vi "x502_recv_out_cycle.vi"() -> ()   [LabVIEW 2010]
uses:
  <vilib>/Waveform/DWDTOps.llb/DWDT Binary U32 to Digital.vi
panel:
  in  "Частота сигнала (Гц)":dbl=50.0 min=1.0 max=500000.0
  in  "Смещение сигнала":dbl min=-5.0 max=5.0 format="%.2f"
  in  "Амплитуда сигнала":dbl=5.0 min=0.0 max=5.0 format="%.2f"
  in  "Подключение по IP":bool
  in  "IP Addr":string="192.168.0.1"
  out "MCU ver":string
  in  "START":bool
  in  "Список устройств USB/PCIe":u16(ring)
  out "Mixed Signal Graph":T1(graph)
  in  "Логические каналы":T2(array[cluster])=[{"PhyCh"=1, "Avg"=1, "Mode"=1, "Range"=0}, {"PhyCh"=2, "Avg"=1, "Mode"=1, "Range"=0}, {"PhyCh"=3, "Avg"=1, "Mode"=1, "Range"=0}] {"Range" items=["10 В", "5 В", "2 В", "1 В", "0.5 В", "0.2 В"]; "Mode" items=["С общей землей", "Дифференциальный", "Измерение нуля"]; "Avg" max=255 step=1; "PhyCh" min=1 max=32 step=1}
  in  "Отображать за время":dbl=250.0 min=10.0 step=1.0
  in  "stop":bool
  out "Установленная частота синхронного ввода DIN":dbl=2.0 min=2.0 max=2000000.0 format="%#_8f"
  in  "Частота синхронного ввода DIN":dbl=20000.0 min=1.0 max=2000000.0 format="%#_8f"
  out "FPGA Ver":string
  in  "Количество каналов":u32=3 min=1 max=3
  out "Установленная частота на канал":dbl=2.0 min=2.0 max=2000000.0 format="%#_8f"
  out "Установленная частота сбора":dbl=2.0 min=2.0 max=2000000.0 format="%#_8f"
  in  "Частота сбора на канал":dbl=2000000.0 min=2.0 max=2000000.0 format="%#_8f"
  in  "Частота сбора (Гц)":dbl=2000000.0 min=2.0 max=2000000.0 format="%#_8f"
  out "PldaVer":u8
  out "Serial":string
  out "Name":string
  # "Информация о плате"
  # "Настройки модуля"
  # "Устанавливаемое"
  # "Установленное"
  # "Вывод на ЦАП"
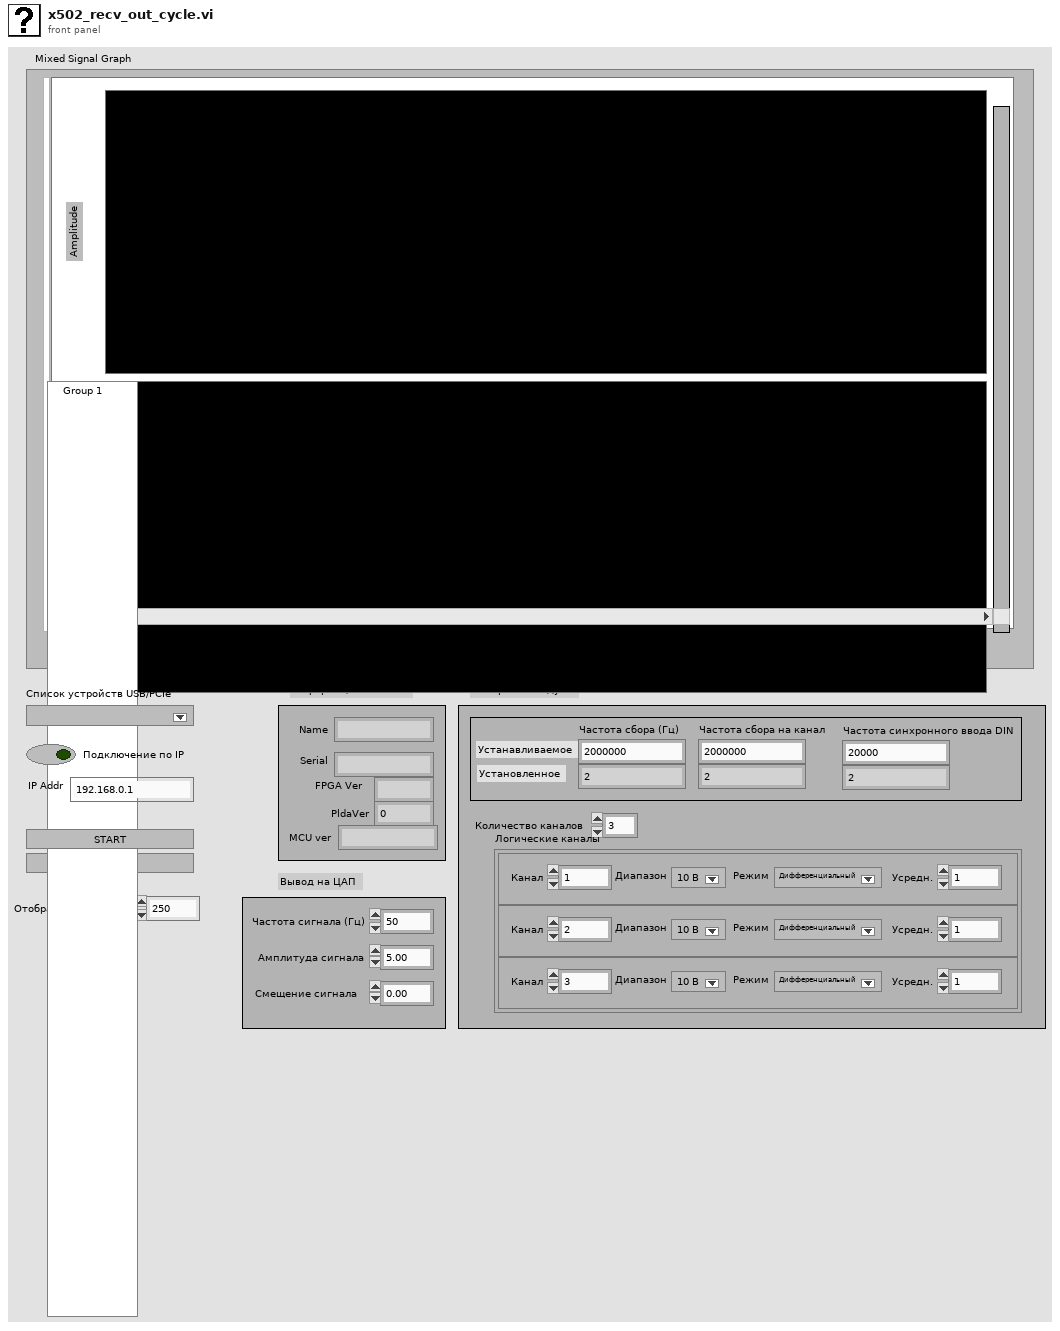
[diagram p1: front panel]
types:
  T1 = cluster{"Dynamic Data Type":dynamicdata, "digital waveform":digitalwaveform}
  T2 = cluster{"PhyCh":u32, "Avg":u32, "Mode":u32, "Range":u32}[]
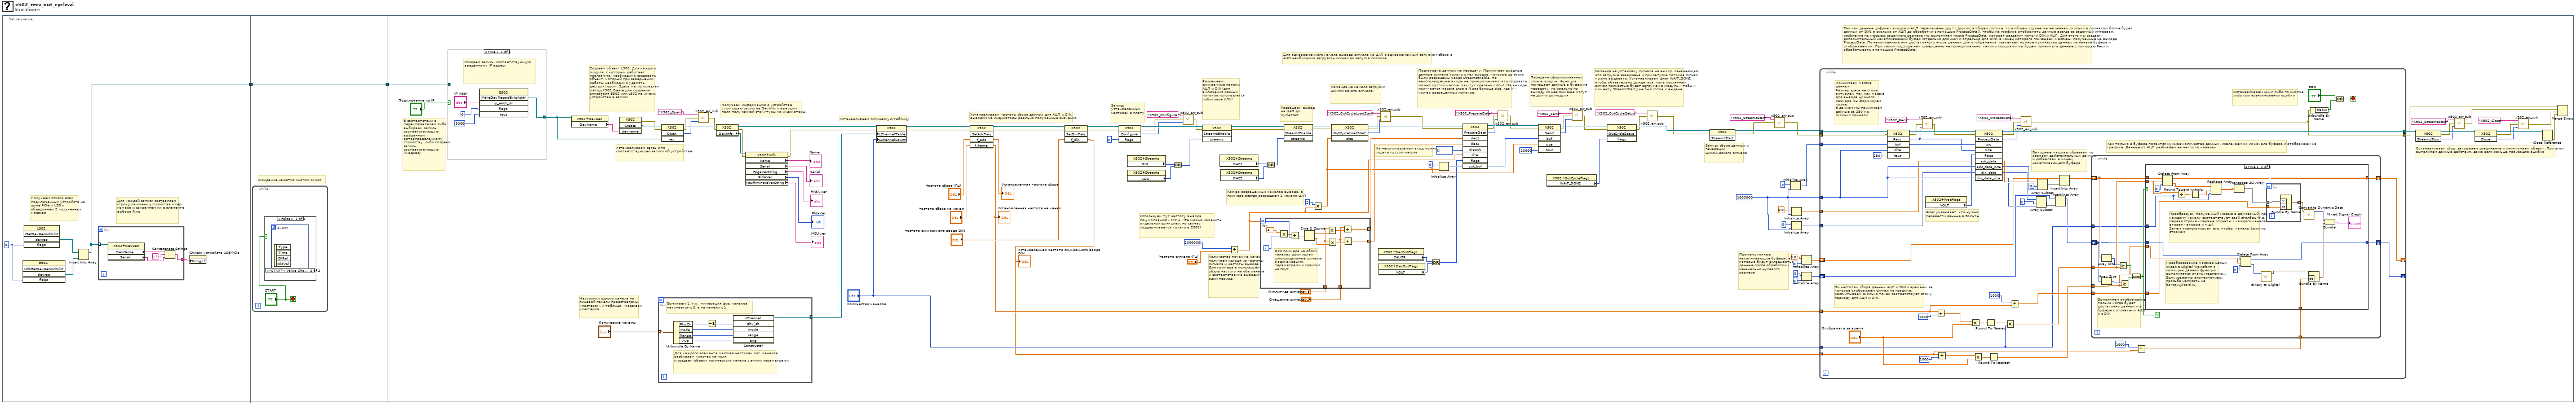
[diagram p0: block diagram]
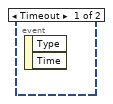
[diagram p2: hidden frame]
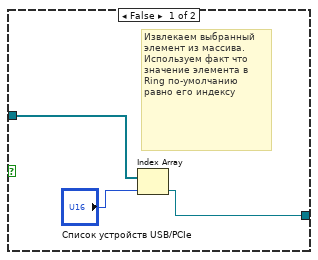
[diagram p5: hidden frame]
diagram:
  n1 = flat-sequence {
    tunnel: [w3] -> w1
    tunnel: [w13] -> w2
    tunnel: w1 -> [w13]
    tunnel: w2 -> [w94]
    frame #0 {
      w5 = 0
      # "Для каждой записи составляем строку из имени устройства и сер. номера и сохраняем их в элементе выбора Ring"
      # "Получаем списко всех подключенных устройств на шине PCIe и USB и объединяем 2 полученных массива"
      n2 = invoke class="E502" method="UsbGetDevRecordsList"("flags"=w5) -> ("devrec"=w6:refnum<k24>[])  [unwired: 4 in, 4 out]
      n3 = invoke class="L502" method="GetDevRecordsList"("flags"=w5) -> ("devrec"=w7:refnum<k24>[])  [unwired: 4 in, 4 out]
      n4 = Insert Into Array(array=w7, new element=w6) -> (w3:refnum<k24>[])  [unwired: 1 in]
      n5 = for {
        tunnel: [w9] -> w4 mode=indexing
        tunnel: w3 -> [w8] mode=indexing
        n6 = property class="X502+DevRec"(reference=w8) -> ("DevName"=w12:string, "Serial"=w10:string)  [unwired: 1 in, 2 out]
        n7 = Concatenate Strings(w12, ", ", w10) -> (w9:string)
      }
      n8 = property on="Список устройств USB/PCIe" class="Ring (strict)"("Strings []"=w4) -> ()  [unwired: 2 in, 2 out]
    }
    frame #1 {
      # "Ожидание нажатия кнопки START"
      n9 = while {
        stop <- "START" stop-if-true
        n10 = case shown="False" "START" {
          frame False {
            n11 = event shown="[1] \"START\": Value Change" {
              selector: _ -> [_ _]
              dyn-events: _ -> [_ _]
              timeout: _ -> [_ _]
              event Timeout {
                n12 = event-data() -> ()  [unwired: 1 in, 2 out]
              }
              event "START": Value Change {
                n13 = event-data() -> ()  [unwired: 1 in, 4 out]
              }
            }
          }
          frame True {
          }
        }
      }
    }
    frame #2 {
      w86 = u32 1000000 ("element")
      # "Останавливаем сбор, закрываем соединение и уничтожаем объект. При этом выполняем данные действия, даже если раньше произошла ошибка"
      # "Команда на установку сигнала на выход, означающая, что загрузка завершена и при запуске потоков сигнал можно выдавать. Устанавливаем флаг WAIT_DONE, чтобы обязательно дождаться, пока посланный сигнал полностью будет загружен в модуль, чтобы к моменту StreamsStart уже был готов к выдаче"
      # "Передача сформированных слов в модуль. Функция помещает данные в буфер на передачу, но раельно по выходу из нее они еще могут не дойти до модуля"
      # "Подготовка данных на передачу. Принимает входные данные сигнала только с тех входов, которые до этого были разрешены через StreamsEnable. На неиспользуемые входы не принципиально, что подовать, можно пустой массив, как тут сделано с dout. На выходе получается массив слов в N раз больше size, где N - кол-во разрешенных потоков."
      # "Команда на начало загрузки циклического сигнала."
      # "Для одновременного начала вывода сигнала на ЦАП с одновременным запуском сбора с АЦП необходимо загрузить сигнал до запуска потоков."
      # "На неиспользуемый вход можно подать пустой массив"
      # "Кол-во разрешенных каналов вывода. В примере всегда разрешаем 2 канала ЦАП"
      # "Количество точек на канал получаем исходя из частоты сигнала и частоты вывода. Для примера в используем обзую частоту на оба канала и соответственно выводим один период"
      # "Используем тут частоту вывода по-умолчанию - 1МГц . (Ее можно изменить отдельной функцией, но сейчас поддерживается только в E502)"
      # "Разрешаем вывод на ЦАП до CycleStart"
      # "Так как данные цифроых входов и АЦП перемешены друг с другом в общем потоке, то в общем случае мы не значем сколько в принятом блоке будет данных от DIN, а сколько от АЦП до обработки с помощью ProcessData(). Чтобы на графике отображать данные всегда за заданный интервал, разбиение на массивы заданного размера мы выполняем после ProcessData, которая разделит потоки DIN и АЦП. Для этого мы создаем дополнительный накапливающий буфер (отдельно для АЦП и отдельно для DIN), в конец которого помещаем массивы, полученные на выходе ProcessData. По накоплению в них достаточного числа данных для отображения  извлекаем нужное количество данных из начала буфера и отображаем их. При таком подходе нам совершенно не принципиально, какими порциями мы будем принимать данные с помощью Recv и обрабатывать с помощью ProcessData."
      # "Промежуточные накапливающие буферы, в которые будут складываться данные после обработки - изначально нулевого размера"
      # "Запуск сбора данных и генерации циклического сигнала"
      # "Разрешаем синхронные потоки АЦП и DIN (для включения разных потоков используется побитовое ИЛИ)"
      # "В соответствии с переключателем либо выбираем запись, соответствующую выбранном автоопределенному стройству, либо создаем запись, соответствующую IP-адресу"
      # "Запись установленных настроек в плату"
      # "Устанавливаем частоты сбора данных для АЦП и DIN,\nвыводим на индикаторы реально полученные значения"
      # "Устанавливаем логическую таблицу"
      # "Настройки одного канала на лицевой панели представлены кластером. А таблица - массивом кластеров."
      # "Создаем объект L502. Для каждого модуля, с которым работает программа, необходимо создавать объект, который при завершении работы необходимо удалять деструктором. Здесь мы используем метод X502.Create для создания описателя E502 или L502 по имени устройства в записи"
      # "Получаем информацию о устройстве \nс помощью свойства DevInfo и выводим\nполя полученной стркутуры на индикаторы"
      # "Устанавливаем связь с по соответствующей записи об устройстве"
      n14 = case shown="True" "Подключение по IP" {
        tunnel: w94 -> [w242 _]
        tunnel: [w240 w243] -> w93
        frame False {
          # "Извлекаем выбранный элемент из массива. Используем факт что значение элемента в Ring по-умолчанию равно его индексу"
          n15 = Index Array(array=w242, index="Список устройств USB/PCIe") -> (element=w240:refnum<k24>)
        }
        frame True {
          # "Создаем запись, соответствующую введенному IP адресу"
          n16 = invoke class="E502" method="MakeDevRecordByIpAddr"("ip_addr_str"="IP Addr", "flags"=0, "tout"=5000) -> ("MakeDevRecordByIpAddr"=w243:refnum<k24>)  [unwired: 3 in, 5 out]
        }
      }
      n17 = property class="X502+DevRec"(reference=w93) -> ("DevName"=w114:string)  [unwired: 1 in, 2 out]
      n18 = invoke class="X502" method="Create"("devname"=w114) -> (error out=w113:errorcluster, "Create"=w115:refnum<k24>)  [unwired: 3 in, 2 out]
      n19 = for {
        tunnel: "Логические каналы" -> [w253] mode=indexing
        tunnel: [w247] -> w131 mode=indexing
        # "Вычитаем 1, т.к.  нумерация физ. каналов начинается с 0, а на панели с 1"
        # "Для каждого элемента массива настроек лог. каналов разбиваем кластер на поля\nи создаем объект логического канала с этими параметрами"
        n20 = Unbundle By Name(w253) -> ("PhyCh"=w252:u32, "Mode"=w250:u32, "Range"=w249:u32, "Avg"=w248:u32)
        n21 = Decrement(x=w252) -> (x-1=w251:u32)
        n22 = constructor class="X502+LChannel"("phy_ch"=w251, "mode"=w250, "range"=w249, "avg"=w248) -> (reference out=w247:refnum<k24>)  [unwired: 3 in, 6 out]
      }
      n23 = invoke class="X502" method="Open"(reference=w115, error in=w113, "rec"=w93) -> (reference out=w116:refnum<k24>, error out=w111:errorcluster, "Open"=w112:i32)  [unwired: 1 in, 1 out]
      n24 = call "x502_err_sub.vi"("Error code"=w112, "error in (no error)"=w111, "Error descr"="X502_Open ") -> ("error out"=w109:errorcluster)
      n25 = property class="X502"(reference=w116, error in=w109) -> (reference out=w117:refnum<k24>, error out=w107:errorcluster, "DevInfo"=w108:refnum<k24>)
      n26 = property class="X502+Info"(reference=w108, error in=w107) -> (error out=w95:errorcluster, "Name"=→"Name":string, "Serial"=→"Serial":string, "FpgaVerString"=→"FPGA Ver":string, "PldaVer"=→"PldaVer":u8, "McuFirmwareVerString"=→"MCU ver":string)  [unwired: 1 out]
      n27 = property class="X502"(reference=w117, error in=w95, "LChannelTable"=w131, "LChannelCount"="Количество каналов") -> (reference out=w118:refnum<k24>, error out=w119:errorcluster)
      n28 = invoke class="X502" method="SetAdcFreq"(reference=w118, error in=w119, "f_adc"="Частота сбора (Гц)", "f_frame"="Частота сбора на канал") -> (reference out=w123:refnum<k24>, error out=w124:errorcluster, "f_adc"=→"Установленная частота сбора":dbl, "f_frame"=w74:dbl)  [unwired: 1 in, 1 out]
      "Установленная частота на канал" <- w74
      n29 = invoke class="X502" method="SetDinFreq"(reference=w123, error in=w124, "f_din"="Частота синхронного ввода DIN") -> (reference out=w128:refnum<k24>, error out=w129:errorcluster, "f_din"=w72:dbl)  [unwired: 1 in, 1 out]
      "Установленная частота синхронного ввода DIN" <- w72
      n30 = invoke class="X502" method="Configure"(reference=w128, error in=w129, "flags"=0) -> (reference out=w130:refnum<k24>, error out=w101:errorcluster, "Configure"=w99:i32)  [unwired: 1 in, 1 out]
      n31 = property class="X502+Streams"() -> ("DIN"=w97:u32)  [unwired: 2 in, 2 out]
      n32 = property class="X502+Streams"() -> ("ADC"=w127:u32)  [unwired: 2 in, 2 out]
      n33 = Or(x=w97, y=w127) -> (x .or. y?=w96:u32)
      n34 = call "x502_err_sub.vi"("Error code"=w99, "error in (no error)"=w101, "Error descr"="X502_Configure ") -> ("error out"=w100:errorcluster)
      n35 = invoke class="X502" method="StreamsEnable"(reference=w130, error in=w100, "streams"=w96) -> (reference out=w66:refnum<k24>, error out=w65:errorcluster)  [unwired: 1 in, 2 out]
      n36 = property class="X502+Streams"() -> ("DAC1"=w68:u32)  [unwired: 2 in, 2 out]
      n37 = property class="X502+Streams"() -> ("DAC2"=w69:u32)  [unwired: 2 in, 2 out]
      n38 = Divide(x=1000000, y="Частота сигнала (Гц)") -> (x/y=w53:dbl)
      n39 = for {
        N: w53 -> [w142]
        tunnel: [w136] -> w57 mode=indexing
        tunnel: [w135] -> w56 mode=indexing
        tunnel: "Амплитуда сигнала" -> [w134]
        tunnel: "Смещение сигнала" -> [w133]
        i -> [w144]
        # "Для примера на обоих каналах формируем синусоидальные сигналы с одинаковыми параметрами и сдвигом на Пи/2"
        n40 = Multiply(x=6.283185307179586, y=w144) -> (x*y=w143:dbl)
        n41 = Divide(x=w143, y=w142) -> (x/y=w141:dbl)
        n42 = Sine & Cosine(0:w141) -> (1:w140:dbl, 2:w138:dbl)
        n43 = Multiply(x=w134, y=w140) -> (x*y=w139:dbl)
        n44 = Multiply(x=w134, y=w138) -> (x*y=w137:dbl)
        n45 = Add(x=w133, y=w139) -> (x+y=w136:dbl)
        n46 = Add(x=w133, y=w137) -> (x+y=w135:dbl)
      }
      n47 = Or(x=w68, y=w69) -> (x .or. y?=w67:u32)
      n48 = invoke class="X502" method="StreamsEnable"(reference=w66, error in=w65, "streams"=w67) -> (reference out=w64:refnum<k24>, error out=w63:errorcluster)  [unwired: 1 in, 2 out]
      n49 = Multiply(x=2, y=w53) -> (x*y=w42:dbl)
      n50 = invoke class="X502" method="OutCycleLoadStart"(reference=w64, error in=w63, "size"=w42) -> (reference out=w58:refnum<k24>, error out=w60:errorcluster, "OutCycleLoadStart"=w61:i32)  [unwired: 1 in, 1 out]
      n51 = property class="X502+DacOutFlags"() -> ("CALIBR"=w50:u32)  [unwired: 2 in, 2 out]
      n52 = property class="X502+DacOutFlags"() -> ("VOLT"=w49:u32)  [unwired: 2 in, 2 out]
      n53 = call "x502_err_sub.vi"("Error code"=w61, "error in (no error)"=w60, "Error descr"="X502_OutCycleLoadStart") -> ("error out"=w55:errorcluster)
      n54 = Or(x=w50, y=w49) -> (x .or. y?=w48:u32)
      n55 = Initialize Array(u32 0 ("element"), w42) -> (w51:u32[])
      n56 = invoke class="X502" method="PrepareData"(reference=w58, error in=w55, "dac1"=w57, "dac2"=w56, "digout"=i32[] [], "size"=w53, "flags"=w48, "out_buf"=w51) -> (reference out=w44:refnum<k24>, error out=w45:errorcluster, "PrepareData"=w46:i32, "out_buf"=w43:u32[])  [unwired: 1 in, 5 out]
      n57 = call "x502_err_sub.vi"("Error code"=w46, "error in (no error)"=w45, "Error descr"="X502_PrepareData") -> ("error out"=w40:errorcluster)
      n58 = invoke class="X502" method="Send"(reference=w44, error in=w40, "buf"=w43, "size"=w42, "tout"=u32 10000 ("element")) -> (reference out=w36:refnum<k24>, error out=w37:errorcluster, "Send"=w38:i32)  [unwired: 1 in, 3 out]
      n59 = property class="X502+OutCycleFlags"() -> ("WAIT_DONE"=w28:u32)  [unwired: 2 in, 2 out]
      n60 = call "x502_err_sub.vi"("Error code"=w38, "error in (no error)"=w37, "Error descr"="X502_Send") -> ("error out"=w35:errorcluster)
      n61 = invoke class="X502" method="OutCycleSetup"(reference=w36, error in=w35, "flags"=w28) -> (reference out=w34:refnum<k24>, error out=w32:errorcluster)  [unwired: 1 in, 2 out]
      n62 = call "x502_err_sub.vi"("error in (no error)"=w32, "Error descr"="X502_OutCycleSetup") -> ("error out"=w31:errorcluster)  [unwired: 1 in]
      n63 = invoke class="X502" method="StreamsStart"(reference=w34, error in=w31) -> (reference out=w76:refnum<k24>, error out=w78:errorcluster)  [unwired: 1 in, 1 out]
      n64 = call "x502_err_sub.vi"("error in (no error)"=w78, "Error descr"="X502_StreamsStart") -> ("error out"=w75:errorcluster)  [unwired: 1 in]
      n65 = Initialize Array(u32 0 ("element"), w86) -> (w87:u32[])
      n66 = Initialize Array(0.0 ("element"), w86) -> (w89:dbl[])
      n67 = Initialize Array(u32 0 ("element"), w86) -> (w88:u32[])
      n68 = Initialize Array(0.0 ("element"), u32 0 ("element")) -> (w91:dbl[])
      n69 = Initialize Array(u32 0 ("element"), u32 0 ("element")) -> (w90:u32[])
      n70 = while {
        tunnel: w76 -> [w198]
        tunnel: w75 -> [w197]
        tunnel: [w196] -> w16
        tunnel: w87 -> [w195]
        shift-right: [w190] -> _
        shift-left: w91 -> [w189]
        shift-right: [w161] -> _
        shift-left: w90 -> [w179]
        tunnel: "Количество каналов" -> [w146]
        tunnel: w74 -> [w162]
        tunnel: w72 -> [w164]
        tunnel: w86 -> [w160]
        tunnel: w88 -> [w159]
        tunnel: w89 -> [w158]
        tunnel: [w147] -> w15
        stop <- w167 stop-if-true
        # "Останавливаем цикл либо по кнопке, либо при возникновении ошибки"
        # "Как только в буфере появится нужное количество данных, извлекаем их из начала буфера и отображаем на графике. Данные от АЦП разбиваем на части по каналам"
        # "По частотам сбора данных АЦП и DIN и времени, за которое отображаем сигнал на графике, рассчитываем сколько точек соответствует этому периоду для АЦП и DIN."
        # "Выходные массивы обрезаем по размеру действительных данных и добавляем в конец накапливающего буфера"
        # "Флаг указывает, что нужно перевести данные в Вольты"
        # "Принимаем массив данных.\nРазмер здесь не столь актуален, так как массив для вывода нужного размера мы формируем позже.\nВ данном мы принимаем данные за 250 мс, сколько приняли"
        n71 = invoke class="X502" method="Recv"(reference=w198, error in=w197, "buf"=w195, "size"=w160, "tout"=u32 250 ("element")) -> (reference out=w186:refnum<k24>, error out=w154:errorcluster, "Recv"=w153:i32, "buf"=w194:u32[])  [unwired: 1 in, 2 out]
        n72 = call "x502_err_sub.vi"("Error code"=w153, "error in (no error)"=w154, "Error descr"="X502_Recv") -> ("error out"=w152:errorcluster)
        n73 = property class="X502+ProcFlags"() -> ("VOLT"=w185:u32)  [unwired: 2 in, 2 out]
        n74 = Divide(x=w162, y=1000) -> (x/y=w177:dbl)
        n75 = Divide(x=w164, y=1000) -> (x/y=w173:dbl)
        n76 = Multiply(x=w177, y="Отображать за время") -> (x*y=w176:dbl)
        n77 = Multiply(x=w173, y="Отображать за время") -> (x*y=w172:dbl)
        n78 = invoke class="X502" method="ProcessData"(reference=w186, error in=w152, "src"=w194, "size"=w153, "flags"=w185, "adc_data"=w158, "adc_data_size"=w160, "din_data"=w159, "din_data_size"=w160) -> (reference out=w196:refnum<k24>, error out=w150:errorcluster, "ProcessData"=w149:i32, "adc_data"=w192:dbl[], "adc_data_size"=w187:u32, "din_data"=w182:u32[], "din_data_size"=w181:u32)  [unwired: 1 in, 3 out]
        n79 = Round To Nearest(number=w176) -> (nearest integer value=w175:dbl)
        n80 = Round To Nearest(number=w172) -> (nearest integer value=w168:dbl)
        n81 = Multiply(x=w175, y=w146) -> (x*y=w169:dbl)
        n82 = Divide(x=u32 1000 ("element"), y=w162) -> (x/y=w157:dbl)
        n83 = call "x502_err_sub.vi"("Error code"=w149, "error in (no error)"=w150, "Error descr"="X502_ProcessData") -> ("error out"=w147:errorcluster)
        n84 = Array Subset(array=w182, index=u32 0 ("element"), length=w181) -> (w180:u32[])
        n85 = Array Subset(array=w192, index=u32 0 ("element"), length=w187) -> (w184:dbl[])
        n86 = Insert Into Array(array=w179, new element=w180) -> (w170:u32[])  [unwired: 1 in]
        n87 = Insert Into Array(array=w189, new element=w184) -> (w188:dbl[])  [unwired: 1 in]
        n88 = Divide(x=u32 1000 ("element"), y=w164) -> (x/y=w156:dbl)
        n89 = while {
          shift-right: [w212] -> w190
          shift-left: w188 -> [w211]
          shift-right: [w202] -> w161
          shift-left: w170 -> [w204]
          tunnel: w169 -> [w209]
          tunnel: w168 -> [w203]
          tunnel: w157 -> [w201]
          tunnel: w156 -> [w200]
          tunnel: w146 -> [w199]
          stop <- w205 continue-if-true
          # "Выполняем отображение только когда будет достаточно данных и в буфере с отсчетами АЦП и с DIN"
          n90 = Array Size(array=w204) -> (size(s)=w208:i32)
          n91 = Array Size(array=w211) -> (size(s)=w210:i32)
          n92 = Greater Or Equal?(x=w210, y=w209) -> (x >= y?=w206:bool)
          n93 = Greater Or Equal?(x=w208, y=w203) -> (x >= y?=w207:bool)
          n94 = And(x=w206, y=w207) -> (x .and. y?=w205:bool)
          n95 = case shown="True" w205 {
            tunnel: [w214 w236] -> w212
            tunnel: w211 -> [w214 w235]
            tunnel: w209 -> [_ w220]
            tunnel: w204 -> [w213 w226]
            tunnel: w203 -> [_ w225]
            tunnel: [w213 w230] -> w202
            tunnel: w201 -> [_ w218]
            tunnel: w200 -> [_ w228]
            tunnel: w199 -> [_ w215]
            frame False {
            }
            frame True {
              # "Преобразуем полученный массив в двумерный, где каждому каналу соответствует свой столбец (т.е. первая строка - первые отсчеты с каждого канала, вторая - вторые и т.д.).\nЗатем транспонируем его, чтобы  каналы были по строкам"
              # "Преобразование массива целых чисел в Digital Waveform с помощью данной функции выполняется очень медленно... Если известны альтернативы, просьба написать на borisov@lcard.ru"
              n96 = Delete From Array(array=w235, length=w220, index=u32 0 ("element")) -> (deleted portion=w219:dbl[], array with subset deleted=w236:dbl[])
              n97 = Divide(x=w220, y=w215) -> (x/y=w224:dbl)
              n98 = Round Toward -Infinity(1:w224) -> (0:w221:dbl)
              n99 = Reshape Array(w219, w221, w215) -> (w223:dbl[][])
              n100 = Transpose 2D Array(2D array=w223) -> (transposed array=w222:dbl[][])
              n101 = Delete From Array(array=w226, length=w225, index=u32 0 ("element")) -> (deleted portion=w232:u32[], array with subset deleted=w230:u32[])
              n102 = call-poly <vilib>:"Binary to Digital.vi"("binary array"=w232) -> ("digital waveform"=w227:digitalwaveform)  [unwired: 9 in, 1 out]
              n103 = for {
                tunnel: w222 -> [w238] mode=indexing
                tunnel: w218 -> [w239]
                tunnel: [w237] -> w217 mode=indexing
                n104 = Bundle By Name("Y"=w238, "dt"=w239) -> (w237:waveform(dbl))  [unwired: 1 in]
              }
              n105 = call "Convert to Dynamic Data"("Array of Waveforms"=w217) -> ("Dynamic Data Type"=w216:dynamicdata)  [unwired: 3 out]
              n106 = Bundle By Name(cluster=w227, "dt"=w228) -> (w231:digitalwaveform)
              n107 = Bundle("Dynamic Data Type"=w216, "digital waveform"=w231) -> (→"Mixed Signal Graph":T1)  [unwired: 1 in]
            }
          }
        }
        n108 = Unbundle By Name(w147) -> ("status"=w148:bool)
        n109 = Or(x="stop", y=w148) -> (x .or. y?=w167:bool)
      }
      n110 = invoke class="X502" method="StreamsStop"(reference=w16) -> (reference out=w26:refnum<k24>, error out=w25:errorcluster, "StreamsStop"=w23:i32)  [unwired: 2 in]
      n111 = call "x502_err_sub.vi"("Error code"=w23, "error in (no error)"=w25, "Error descr"="X502_StreamsStop") -> ("error out"=w17:errorcluster)
      n112 = invoke class="X502" method="Close"(reference=w26) -> (reference out=w27:refnum<k24>, error out=w21:errorcluster, "Close"=w20:i32)  [unwired: 2 in]
      n113 = call "x502_err_sub.vi"("Error code"=w20, "error in (no error)"=w21, "Error descr"="X502_Close") -> ("error out"=w18:errorcluster)
      n114 = Close Reference(reference=w27) -> (error out=w19:errorcluster)  [unwired: 1 in]
      n115 = Merge Errors(w15, w17, w18, w19) -> ()  [unwired: 1 out]
    }
  }
